vi "TDMS Rename Run.vi"(6 "Run Number":i32, 8 "error in (no error)":errorcluster, 9 "Run Name (\"\")":string, 10 "Run to Rename (\"\")":string, 11 "TDMS File Ref In":refnum<k34>) -> (0 "error out":errorcluster, 3 "TDMS File Ref Out":refnum<k34>)   [LabVIEW 2011]
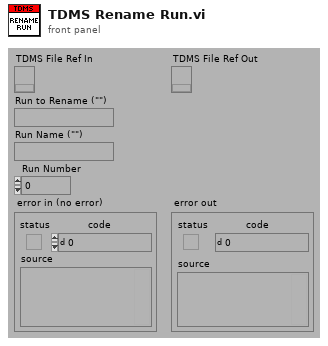
[diagram p1: front panel]
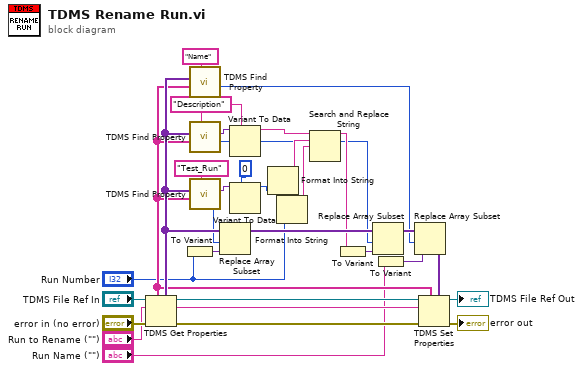
[diagram p0: block diagram]
diagram:
  w24 = "Description" ("Property Name")
  n1 = TDMS Get Properties(8:"error in (no error)", 10:"Run to Rename (\"\")", 11:"TDMS File Ref In") -> (0:w10:errorcluster, 2:w8:string, 3:w11:refnum<k34>, 4:w31:variant[], 6:w9:string[])  [unwired: 3 in, 1 out]
  n2 = To Variant(anything="Run Number") -> (Variant=w28:variant)
  n3 = call "TDMS Find Property.vi"("Property Name"="Name", "Property Names"=w9, "Property Values"=w31) -> ("Index"=w12:i32)  [unwired: 4 in, 1 out]
  n4 = call "TDMS Find Property.vi"("Property Name"=w24, "Property Names"=w9, "Property Values"=w31) -> ("Index"=w16:i32, "Property Value"=w29:variant)  [unwired: 4 out]
  n5 = call "TDMS Find Property.vi"("Property Name"="Test_Run", "Property Names"=w9, "Property Values"=w31) -> ("Index"=w27:i32, "Property Value"=w22:variant)  [unwired: 4 out]
  n6 = Replace Array Subset(array=w31, new element=w28, index=w27) -> (w25:variant[])
  n7 = Variant To Data(type=w24, Variant=w29) -> (data=w23:string)  [unwired: 1 in, 1 out]
  n8 = Variant To Data(type=0, Variant=w22) -> (data=w20:i32)  [unwired: 1 in, 1 out]
  n9 = Format Into String(w20) -> (resulting string=w19:string)  [unwired: 3 in, 1 out]
  n10 = Format Into String("Run Number") -> (resulting string=w18:string)  [unwired: 3 in, 1 out]
  n11 = Search and Replace String(input string=w23, search string=w19, replace string=w18) -> (result string=w17:string)  [unwired: 5 in, 3 out]
  n12 = To Variant(anything=w17) -> (Variant=w26:variant)
  n13 = Replace Array Subset(array=w25, new element=w26, index=w16) -> (w14:variant[])
  n14 = To Variant(anything="Run Name (\"\")") -> (Variant=w15:variant)
  n15 = Replace Array Subset(array=w14, new element=w15, index=w12) -> (w32:variant[])
  n16 = TDMS Set Properties(5:w32, 7:w9, 8:w10, 10:w8, 11:w11) -> (0:→"error out":errorcluster, 3:→"TDMS File Ref Out":refnum<k34>)  [unwired: 1 in, 2 out]
